vi "Set Attr Filter.vi"(8 "error in (no error)":errorcluster, 10 "Attr Filter":string, 11 "Camera Settings Dialog in":refnum<class "Camera Settings Dialog.lvclass">) -> (0 "error out":errorcluster, 3 "Camera Settings Dialog out":refnum<class "Camera Settings Dialog.lvclass">)   [LabVIEW 2020, in "Camera Settings Dialog UI.lvlib" / "Camera Settings Dialog.lvclass"]
uses:
  Camera Settings Dialog.lvclass
  Camera Settings Dialog.lvclass/Camera Settings Dialog.ctl
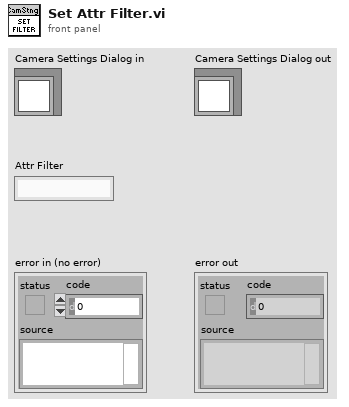
[diagram p1: front panel]
types:
  T1 = typedef "Camera Attribute Info.ctl" = cluster{"Attribute Type":string, "Readable":bool, "Writable":bool, "Attribute Name":string, "DisplayName":string, "Units":string, "Tooltip":string, "ValueString":string, "MaxDBL":dbl, "MaxI64":i64, "MaxString":string, "MaxU32":u32, "MinDBL":dbl, "MinI64":i64, "MinString":string, "MinU32":u32, "ValueBool":bool, "ValueDBL":dbl, "ValueI64 ":i64, "ValueString":string, "ValueU32":u32, "IncDBL":dbl, "IncU32":u32, "IncI64":i64, "EnumStrings":string[], "EnumValues":u32[]}
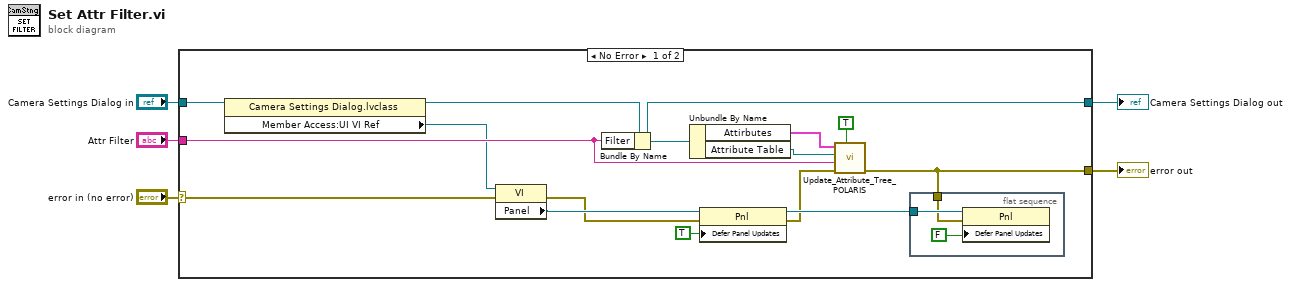
[diagram p0: block diagram]
diagram:
  n1 = case shown="No Error" "error in (no error)" {
    selector: "error in (no error)" -> [w8 w24]
    tunnel: [w6 w24] -> w4
    tunnel: [w16 w23] -> w2
    tunnel: "Camera Settings Dialog in" -> [w19 w23]
    tunnel: "Attr Filter" -> [w17 _]
    frame No Error {
      n2 = property class="Camera Settings Dialog.lvclass"(reference=w19) -> (reference out=w13:refnum<class "Camera Settings Dialog.lvclass">, "Member Access:UI VI Ref"=w10:refnum<vi>)  [unwired: 1 in, 1 out]
      n3 = property class="VI"(reference=w10) -> ("Panel"=w9:refnum<vi>)  [unwired: 1 in, 2 out]
      n4 = Bundle By Name(cluster=w13, "Filter"=w17) -> (w16:refnum<class "Camera Settings Dialog.lvclass">)
      n5 = Unbundle By Name(w16) -> ("Attirbutes"=w15:T1[], "Attribute Table"=w14:refnum<vi>)
      n6 = property class="Pnl"(reference=w9, error in=w8, "Defer Panel Updates"=TRUE) -> (reference out=w12:refnum<vi>, error out=w7:errorcluster)
      n7 = call "Update_Attribute_Tree_POLARIS.vi"("Flush Tree?"=TRUE, "error in"=w7, "Filter"=w17, "Tree Control In"=w14, "Attribute Information Array"=w15) -> ("error out"=w6:errorcluster)  [unwired: 3 in]
      n8 = flat-sequence {
        tunnel: w12 -> [w22]
        tunnel: w6 -> [w20]
        frame #0 {
          n9 = property class="Pnl"(reference=w22, error in=w20, "Defer Panel Updates"=FALSE) -> ()  [unwired: 2 out]
        }
      }
    }
    frame Error {
    }
  }
  "error out" <- w4
  "Camera Settings Dialog out" <- w2
